vi "Read Block.vi"(8 "error in (no error)":errorcluster, 11 "VISA resource name in":refnum<visa-resource-name>) -> (0 "error out":errorcluster, 2 "Data":string, 3 "VISA resource name":refnum<visa-resource-name>)   [LabVIEW 2023, in "CTI-Visa.lvlib"]
uses:
  CTI-Visa.lvlib
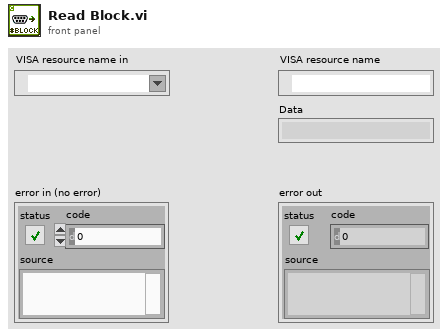
[diagram p1: front panel]
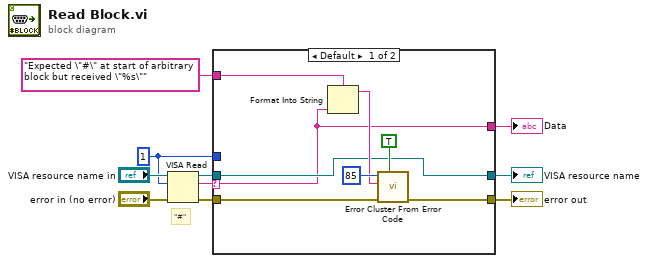
[diagram p0: block diagram]
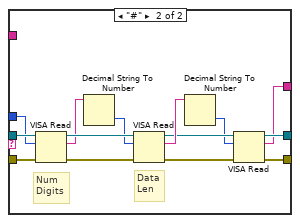
[diagram p2: hidden frame]
diagram:
  w4 = u32 1 ("byte count")
  # "\"#\""
  n1 = VISA Read(VISA resource name="VISA resource name in", byte count=w4, error in (no error)="error in (no error)") -> (VISA resource name out=w6:refnum<visa-resource-name>, read buffer=w7:string, error out=w5:errorcluster)  [unwired: 1 out]
  n2 = case shown="Default" w7 {
    selector: w7 -> [w11 _]
    tunnel: w6 -> [w13 w32]
    tunnel: w5 -> [w18 w31]
    tunnel: w4 -> [_ w30]
    tunnel: [w14 w20] -> w10
    tunnel: [w13 w21] -> w3
    tunnel: [w11 w19] -> w2
    tunnel: "Expected \"#\" at start of arbitrary block but received \"%s\"" -> [w12 _]
    frame Default {
      n3 = Format Into String(format string=w12, w11) -> (resulting string=w16:string)  [unwired: 2 in, 1 out]
      n4 = call <vilib>:"Error Cluster From Error Code.vi"("show call chain? (False)"=TRUE, "error in (no error)"=w18, "error message (\"\")"=w16, "error code (0)"=85) -> ("error out"=w14:errorcluster)  [unwired: 5 in]
    }
    frame "#" {
      # "Data\nLen"
      # "Num\nDigits"
      n5 = VISA Read(VISA resource name=w32, byte count=w30, error in (no error)=w31) -> (VISA resource name out=w29:refnum<visa-resource-name>, read buffer=w27:string, error out=w28:errorcluster)  [unwired: 1 out]
      n6 = Decimal String To Number(string=w27) -> (number=w26:i32)  [unwired: 2 in, 1 out]
      n7 = VISA Read(VISA resource name=w29, byte count=w26, error in (no error)=w28) -> (VISA resource name out=w24:refnum<visa-resource-name>, read buffer=w25:string, error out=w23:errorcluster)  [unwired: 1 out]
      n8 = Decimal String To Number(string=w25) -> (number=w22:i32)  [unwired: 2 in, 1 out]
      n9 = VISA Read(VISA resource name=w24, byte count=w22, error in (no error)=w23) -> (VISA resource name out=w21:refnum<visa-resource-name>, read buffer=w19:string, error out=w20:errorcluster)  [unwired: 1 out]
    }
  }
  "VISA resource name" <- w3
  "error out" <- w10
  "Data" <- w2
